vi "Discard.vi"(8 "error in":errorcluster, 10 "index":i32, 11 "Machine In":refnum<visa-resource-name>) -> (0 "error out":errorcluster, 3 "Machine Out":refnum<visa-resource-name>)   [LabVIEW 2018]
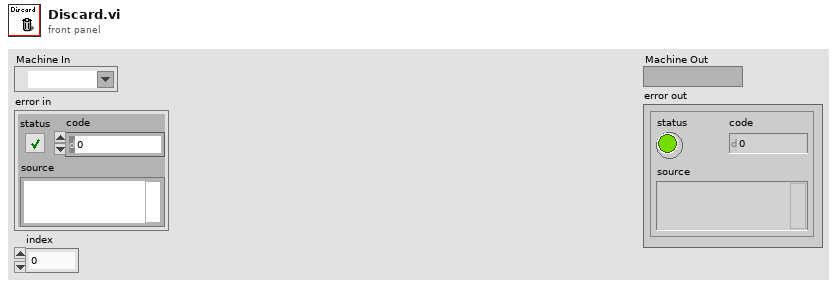
[diagram p1: front panel]
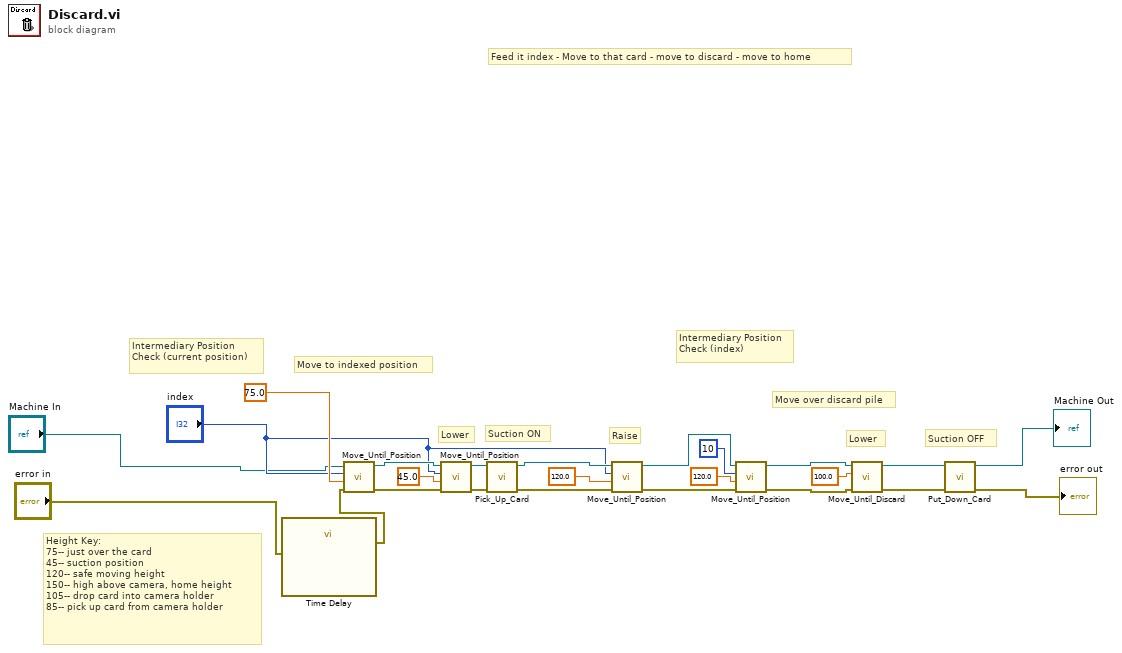
[diagram p0: block diagram]
diagram:
  # "Height Key:\n75-- just over the card\n45-- suction position\n120-- safe moving height\n150-- high above camera, home height\n105-- drop card into camera holder\n85-- pick up card from camera holder"
  # "Suction ON"
  # "Intermediary Position Check (index)"
  # "Intermediary Position Check (current position)"
  # "Raise"
  # "Lower"
  # "Lower"
  # "Move to indexed position"
  # "Suction OFF"
  # "Move over discard pile"
  # "Feed it index - Move to that card - move to discard - move to home"
  n1 = call "Time Delay"("error in (no error)"="error in") -> ("error out"=w10:errorcluster)  [unwired: 10 in]
  n2 = call "Move_Until_Position.vi"("error in (no error)"=w10, "Z-Position"=75.0, "index"="index", "VISA Refnum in"="Machine In") -> ("error out"=w23:errorcluster, "VISA Refnum out"=w24:refnum<visa-resource-name>)  [unwired: 6 in]
  n3 = call "Move_Until_Position.vi"("error in (no error)"=w23, "Z-Position"=45.0, "index"="index", "VISA Refnum in"=w24) -> ("error out"=w14:errorcluster, "VISA Refnum out"=w15:refnum<visa-resource-name>)  [unwired: 6 in]
  n4 = call "Pick_Up_Card.vi"("error in"=w14, "VISA Refnum in"=w15) -> ("error out"=w12:errorcluster, "Machine Out"=w13:refnum<visa-resource-name>)  [unwired: 6 in]
  n5 = call "Move_Until_Position.vi"("error in (no error)"=w12, "Z-Position"=120.0, "index"="index", "VISA Refnum in"=w13) -> ("error out"=w16:errorcluster, "VISA Refnum out"=w17:refnum<visa-resource-name>)  [unwired: 6 in]
  n6 = call "Move_Until_Position.vi"("error in (no error)"=w16, "Z-Position"=120.0, "index"=10, "VISA Refnum in"=w17) -> ("error out"=w3:errorcluster, "VISA Refnum out"=w4:refnum<visa-resource-name>)  [unwired: 6 in]
  n7 = call "Move_Until_Discard.vi"("error in (no error)"=w3, "Desired Height"=100.0, "VISA Refnum in"=w4) -> ("error out"=w11:errorcluster, "VISA Refnum out"=w20:refnum<visa-resource-name>)  [unwired: 7 in]
  n8 = call "Put_Down_Card.vi"("error in"=w11, "VISA Refnum in"=w20) -> ("error out"=→"error out":errorcluster, "Machine Out"=→"Machine Out":refnum<visa-resource-name>)  [unwired: 7 in]
